vi "zigZagVelPlanning.vi"(5 "delta interval":dbl, 6 "test number":i32, 7 "start?":bool=TRUE, 8 "error in (no error)":errorcluster, 9 "Dest_array":T3(array[cluster]), 10 "id":i32, 11 "Game in":refnum<class "Game.lvclass">) -> (0 "error out":errorcluster, 1 "replace":bool, 2 "TestTeam":refnum<class "Ally.lvclass">, 3 "Game out":refnum<class "Game.lvclass">, 4 "velocityPlanningState":T1={"est_vel"=0.0, "dist_to_(Dest/L)"=0.0, "V0_model"=0.0, "max_dist_to_break"=0.0, "v_sent"=0.0, "traj_state"=enum."replace"})   [LabVIEW 2023, in "Game.lvclass"]
uses:
  Game.lvclass
  Ally_class/Ally.lvclass
  C:/Users/lucio/Desktop/roboime/SSL_AI/Team_class/Team.lvclass
  VelocityPlanningTest/Controls/velocityPlanningState.ctl
  VelocityPlanningTest/Controls/trajectoryState.ctl
  <vilib>/Analysis/coordinate.llb/Angle Units.ctl
  Game.lvclass/Game.ctl
  Team_class/Team.lvclass/Team.ctl
  Robot_class/Robot.lvclass/Robot.ctl
  Object_class/Object.lvclass/Object.ctl
  Navigation/Controls/typeOfUse.ctl
  Communication_class/Paths/grSim Packet Command UDP Test Folder/grSim/grSim RobotReplacement.ctl
  <vilib>/Analysis/coordinate.llb/Wrap Angle (scalar).vi
  <vilib>/Analysis/_algsub.llb/Real Vector Norm.vi
  Robot_class/Write v_tang.vi
  Robot_class/Write v_norm.vi
  Robot_class/Write v_ang.vi
  Read AllyRef.vi
  Read NewParameters.vi
  Team_class/Read RobotRef.vi
  Robot_class/Read est_v_ang.vi
  Robot_class/Read est_v_norm.vi
  Robot_class/Read est_v_tang.vi
  Object_class/Read x.vi
  Object_class/Read y.vi
  Robot_class/Read orientation.vi
  Robot_class/Write dest_x.vi
  Robot_class/Write dest_y.vi
  Robot_class/Write dest_orientation.vi
  Robot_class/Read dest_x.vi
  Robot_class/Read dest_y.vi
  Robot_class/Read dest_orientation.vi
  Team_class/Write RobotRef.vi
  Robot_class/Robot.lvclass
  C:/Users/lucio/Desktop/roboime/SSL_AI/Object_class/Object.lvclass
  Utilities_class/Utilities.lvclass
  <vilib>/Analysis/NI_AALPro.lvlib
  <vilib>/Analysis/NI_AAL_Angle.lvlib
panel:
  out "appended array":bool[](array[boolean])
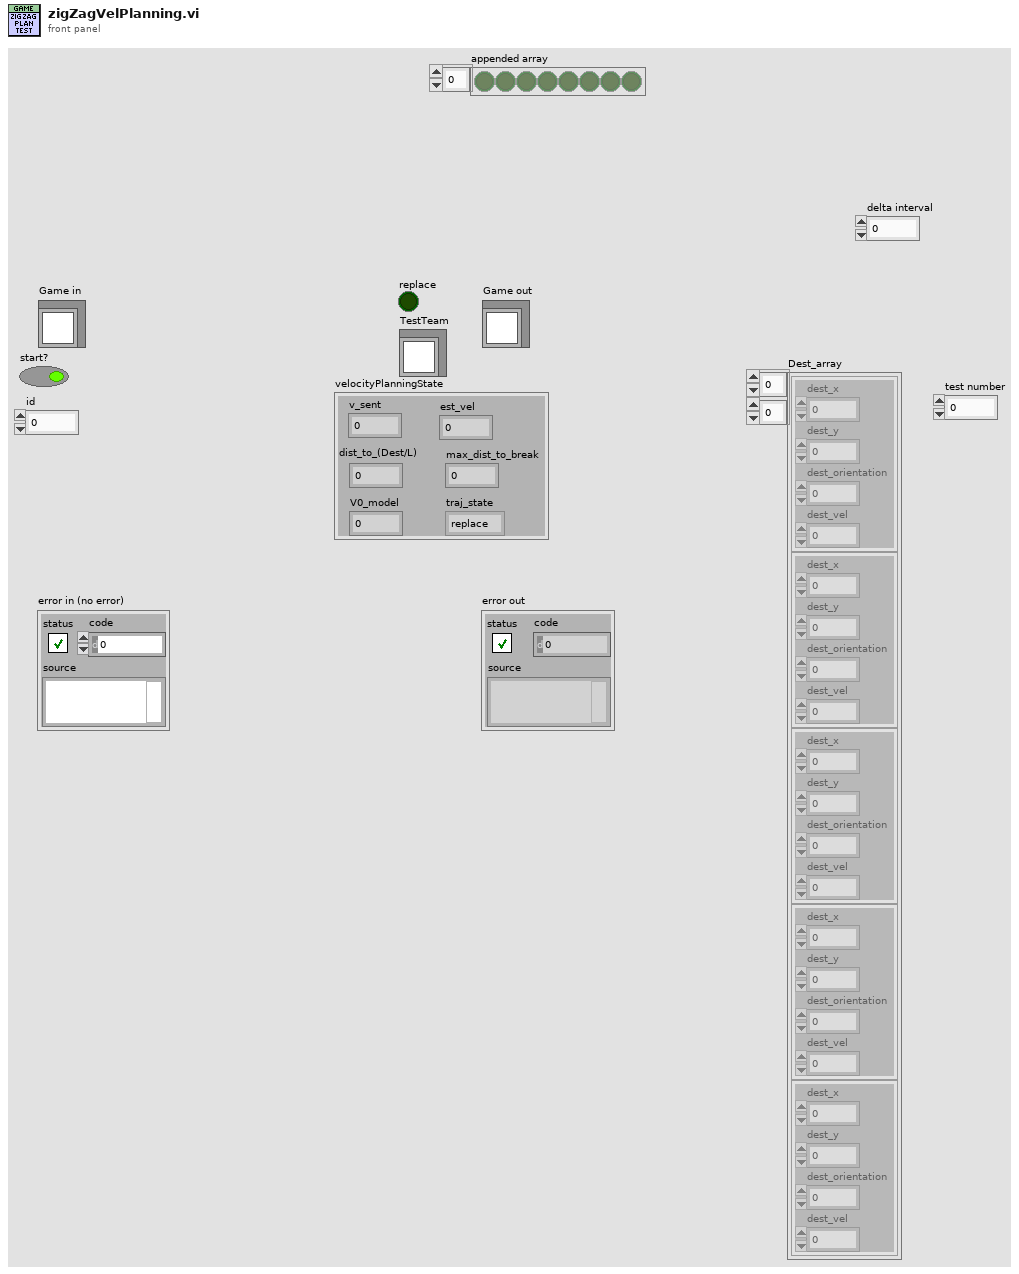
[diagram p1: front panel]
types:
  T1 = typedef "velocityPlanningState.ctl" = cluster{"est_vel":dbl, "dist_to_(Dest/L)":dbl, "V0_model":dbl, "max_dist_to_break":dbl, "v_sent":dbl, "traj_state":T2}
  T2 = typedef "trajectoryState.ctl" = enum16{"stop", "replace", "circle", "line", "turn"}
  T3 = cluster{"dest_x":dbl, "dest_y":dbl, "dest_orientation":dbl, "dest_vel":dbl}[][]
  T4 = cluster{"dest_x":dbl, "dest_y":dbl, "dest_orientation":dbl, "dest_vel":dbl}[]
  T5 = typedef "grSim RobotReplacement.ctl" = cluster{"x":dbl, "y":dbl, "dir(degree)":dbl, "yellowteam":bool, "id":u32}
  T6 = typedef "typeOfUse.ctl" = enum16{"Navigation", "ZigZag", "grSimTest"}
  T7 = typedef "NI_AAL_Angle.lvlib/Angle Units.ctl" = i32
  T8 = typedef "NewParameters.ctl" = cluster{"PenaltyDistance":dbl, "DistanceAttackerToBackBall":dbl, "Division":enum16{"Div B", "Div A"}, "DistanceToAvoidyEnemyRobot":dbl, "BallPlacementDistance":dbl, "DisatanceBehindBallToStealBall":dbl, "MaxDistanceToPositionKickoff":dbl, "BlockEnemyTarget":bool, "MaxStopVAng":dbl, "DistanceMarkerToEnemy":dbl, "IgnoreDribblerContact":bool, "DistanceToBeginEnemyPosession":dbl, "GoToBallWhenEnemyNotMoving":bool, "EnemyDistanceToReduceVelocity":dbl, "TurnOnEnemyDistanceToReduceVelocity":bool, "EnemyDistanceToShootOutBall":dbl, "DefenseKickBall":bool, "MoreKickToGoal? (0-0.3)":dbl, "ChipKickInEnemyField":bool, "ShootOutRobotId":dbl, "FieldLenghtDenominatorInShootOut":dbl, "AdjustPositionInBallPlacement":bool, "PowerGodPass":dbl, "VelocityAbortEnemyPos":dbl, "MaxDistToBeginPass":dbl, "MinDistToBeginPass":dbl, "VelocityInDirects":dbl, "BadDribblerIDs":i32[], "NewKickToDistanceAroundBall":dbl, "PowerAvoidColisionMarker":dbl, "DistanceToAvoidColisionMarker":dbl, "AvoidBallKick":dbl, "DistanceTryKick":dbl, "SuicideKickDIstance":dbl, "AdjustFirstKickDistance":dbl, "AvoidAimLessKick":dbl, "DistanceToAvoidyEnemyShootRobot ":dbl, "NumberOfMarkers":dbl, "PotField":bool, "PIDLateral":bool, "MinDistanceFirstKickX":dbl, "MinDistanceFirstKickY":dbl, "FractionOfDistToTouchGround\nAfterChipKick":dbl, "FractionOfKickxWhen\nComposedWithKickz":dbl, "Style":T9, "MoveInTurnState":bool, "DistFromEnemyToConsider\nMoveInTurnState":dbl, "CascadePID":bool, "TurnAroundParameters":cluster{"Radius":dbl, "Multiplier":dbl, "ChordAngle":dbl}, "SafeDriveVel":dbl, "DistanceToGoToBackBall":dbl, "minDistanceToNotFinish\nEnemyPossession":dbl, "OneTouchShot":cluster{"angleFactor":dbl, "maxAngle":dbl, "Attack":bool, "Defense":bool}, "OpenAngleToGoal":cluster{"minAngle":dbl, "maxAngle":dbl, "minEvaluation":dbl}, "ShotInterception":cluster{"shotSpeed":dbl, "minEnemySpeed":dbl, "maxEnemySpeed":dbl, "minEvaluation":dbl}, "AllyTeamArray":T10[], "maxDefendersNumber":i32, "Zone":cluster{"GuardPositionArray":dbl[][], "ZoneMidField":dbl[], "CenterForwardWidth":dbl}, "MinEvaluationToShoot":dbl, "PassInterception":cluster{"maxPassSpeed":dbl, "minPassSpeed":dbl, "minEnemySpeed":dbl, "chipPassDistance":dbl, "chipPassEvaluation":dbl, "minEvaluation":dbl, "maxEnemySpeed":dbl}, "PassDistance":cluster{"maxDistance":dbl, "minDistance":dbl}, "receiverSpeed":dbl, "maxBallSpeed":dbl, "slackTime":dbl, "Turning radius":dbl, "Turning v_ang":dbl, "AlignError":cluster{"Distance":dbl, "Orientation":dbl, "V_norm(m/s)":dbl, "V_ang (rad/s)":dbl}, "RobotRadius":dbl, "KickerDistance":dbl, "keeper angle  to cover goalpost":dbl}
  T9 = typedef "Style.ctl" = enum16{"Insanity", "Offensive", "Defensive"}
  T10 = typedef "AllyTeam.ctl" = enum16{"Keeper", "Defender", "Attacker"}
  T11 = cluster{"dest_x":dbl, "dest_y":dbl, "dest_orientation":dbl, "dest_vel":dbl}
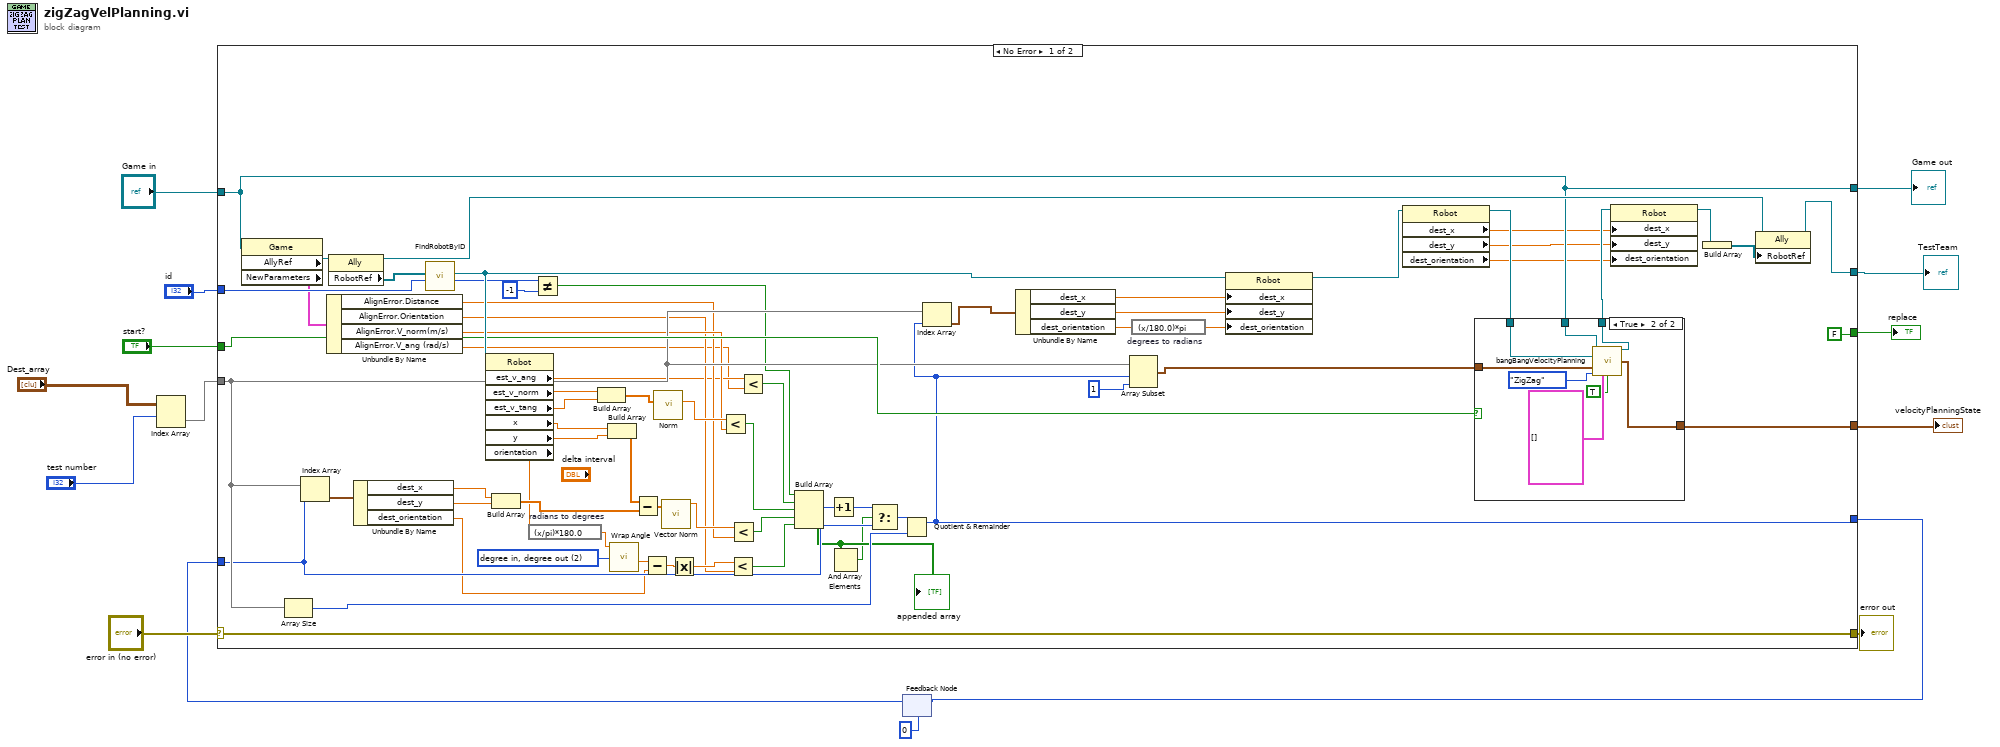
[diagram p0: block diagram]
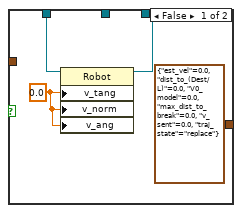
[diagram p2: hidden frame]
diagram:
  n1 = Index Array(array="Dest_array", index (row)="test number") -> (element=w1:T4)  [unwired: 1 in]
  n2 = feedback #1(0) -> (w8:i32)
  n3 = case shown="No Error" "error in (no error)" {
    selector: "error in (no error)" -> [w82 w95]
    tunnel: [w82 w95] -> w14
    tunnel: "Game in" -> [w74 _]
    tunnel: [w74 _] -> w12
    tunnel: w1 -> [w44 _]
    tunnel: [w73 _] -> w11
    tunnel: [w72 _] -> w10
    tunnel: "id" -> [w71 _]
    tunnel: w8 -> [w39 _]
    tunnel: [w43 _] -> w6
    tunnel: [FALSE _] -> w5
    tunnel: "start?" -> [w60 _]
    frame No Error {
      w24 = T7 2 items=["radian in, radian out", "radian in, degree out", "degree in, degree out", "degree in, radian out"] ("angle units")
      n4 = property class="Game"(reference=w74) -> ("AllyRef"=w81:refnum<class "Ally.lvclass">, "NewParameters"=w32:T8)  [unwired: 1 in, 2 out]
      n5 = Array Size(array=w44) -> (size(s)=w45:i32)
      n6 = Index Array(array=w44, index=w39) -> (element=w46:T11)
      n7 = Unbundle By Name(w32) -> ("AlignError.Distance"=w29:dbl, "AlignError.Orientation"=w30:dbl, "AlignError.V_norm(m/s)"=w31:dbl, "AlignError.V_ang (rad/s)"=w27:dbl)
      n8 = property class="Ally"(reference=w81) -> (reference out=w78:refnum<class "Ally.lvclass">, "RobotRef"=w80:refnum<class "Robot.lvclass">[])  [unwired: 1 in, 1 out]
      n9 = Unbundle By Name(w46) -> ("dest_x"=w70:dbl, "dest_y"=w69:dbl, "dest_orientation"=w26:dbl)
      n10 = call "FindRobotByID.vi"("id"=w71, "RobotRef"=w80) -> ("index"=w58:i32, "Robot"=w66:refnum<class "Robot.lvclass">)  [unwired: 6 in, 2 out]
      n11 = property class="Robot"(reference=w66) -> ("est_v_ang"=w28:dbl, "est_v_norm"=w36:dbl, "est_v_tang"=w35:dbl, "x"=w65:dbl, "y"=w64:dbl, "orientation"=w38:dbl)  [unwired: 1 in, 2 out]
      n12 = Build Array(w70, w69) -> (w68:dbl[])
      n13 = expression code="(x/pi)*180.0" "radians to degrees"(w38) -> (w25:dbl)
      n14 = Not Equal?(x=w58, y=-1) -> (x != y?=w22:bool)
      n15 = Build Array(w36, w35) -> (w34:dbl[])
      n16 = Build Array(w65, w64) -> (w63:dbl[])
      n17 = call-poly <vilib>:"Wrap Angle.vi"("angle units"=w24, "angle in"=w25) -> ("angle out"=w23:dbl)  [unwired: 8 in, 1 out]
      n18 = Subtract(x=w63, y=w68) -> (x-y=w67:dbl[])
      n19 = Subtract(x=w23, y=w26) -> (x-y=w37:dbl)
      n20 = call "Norm.vi"("2D vector"=w34) -> ("Modulo"=w33:dbl)  [unwired: 8 in, 2 out]
      n21 = call-poly <vilib>:"Vector Norm.vi"("Input Vector"=w67) -> ("norm"=w62:dbl)  [unwired: 9 in, 1 out]
      n22 = Absolute Value(x=w37) -> (abs(x)=w55:dbl)
      n23 = Less?(x=w33, y=w31) -> (x < y?=w20:bool)
      n24 = Less?(x=w55, y=w30) -> (x < y?=w18:bool)
      n25 = Less?(x=w62, y=w29) -> (x < y?=w19:bool)
      n26 = Less?(x=w28, y=w27) -> (x < y?=w21:bool)
      n27 = Build Array(w22, w21, w20, w19, w18) -> (w17:bool[])
      "appended array" <- w17
      n28 = Increment(x=w39) -> (x+1=w40:i32)
      n29 = And Array Elements(Boolean array=w17) -> (logical AND=w16:bool)
      n30 = Select(t=w40, s=w16, f=w39) -> (s? t:f=w59:i32)
      n31 = Quotient & Remainder(x=w59, y=w45) -> (x-y*floor(x/y)=w43:i32)  [unwired: 1 out]
      n32 = Index Array(array=w44, index=w43) -> (element=w41:T11)
      n33 = Unbundle By Name(w41) -> ("dest_x"=w77:dbl, "dest_y"=w76:dbl, "dest_orientation"=w54:dbl)
      n34 = Array Subset(array=w44, index=w43, length=1) -> (w56:T4)
      n35 = expression code="(x/180.0)*pi" "degrees to radians"(w54) -> (w75:dbl)
      n36 = property class="Robot"(reference=w66, "dest_x"=w77, "dest_y"=w76, "dest_orientation"=w75) -> (reference out=w51:refnum<class "Robot.lvclass">)  [unwired: 1 in, 1 out]
      n37 = property class="Robot"(reference=w51) -> (reference out=w50:refnum<class "Robot.lvclass">, "dest_x"=w49:dbl, "dest_y"=w48:dbl, "dest_orientation"=w47:dbl)  [unwired: 1 in, 1 out]
      n38 = case shown="True" w60 {
        tunnel: [w84 w94] -> w53
        tunnel: w50 -> [w85 w92]
        tunnel: w74 -> [_ w91]
        tunnel: [T1 {"est_vel"=0.0, "dist_to_(Dest/L)"=0.0, "V0_model"=0.0, "max_dist_to_break"=0.0, "v_sent"=0.0, "traj_state"=enum."replace"} ("velocityPlanningState") w90] -> w73
        tunnel: w56 -> [_ w87]
        frame False {
          w83 = 0.0
          n39 = property class="Robot"(reference=w85, "v_tang"=w83, "v_norm"=w83, "v_ang"=w83) -> (reference out=w84:refnum<class "Robot.lvclass">)  [unwired: 1 in, 1 out]
        }
        frame True {
          n40 = call "bangBangVelocityPlanning.vi"("Game"=w91, "Robot in"=w92, "Dest_array"=w87, "type_of_use"=typeOfUse."ZigZag", "robots_test"=T5[] [], "start"=TRUE) -> ("Robot out"=w94:refnum<class "Robot.lvclass">, "velocityPlanningState"=w90:T1)  [unwired: 7 in, 1 out]
        }
      }
      n41 = property class="Robot"(reference=w53, "dest_x"=w49, "dest_y"=w48, "dest_orientation"=w47) -> (reference out=w52:refnum<class "Robot.lvclass">)  [unwired: 1 in, 1 out]
      n42 = Build Array(w52) -> (w79:refnum<class "Robot.lvclass">[])
      n43 = property class="Ally"(reference=w78, "RobotRef"=w79) -> (reference out=w72:refnum<class "Ally.lvclass">)  [unwired: 1 in, 1 out]
    }
    frame Error {
    }
  }
  "error out" <- w14
  "Game out" <- w12
  "TestTeam" <- w10
  "velocityPlanningState" <- w11
  "replace" <- w5
  n44 = feedback-in #1(w6) -> ()
